vi "raspberry pi red.vi"() -> ()   [LabVIEW 2018]
panel:
  out "Numeric 2":dbl
  out "Waveform Chart 2":dbl(graph)
  out "Humedad":dbl(slide) scale=0.0..100.0
  out "Numeric":dbl
  out "Lectura Raspberry PI":string
  in  "Direcciòn IP":string
  in  "Puerto":i32
  in  "stop":bool
  out "Waveform Chart":dbl(graph)
  out "Temperatura °C":dbl(slide) scale=0.0..100.0
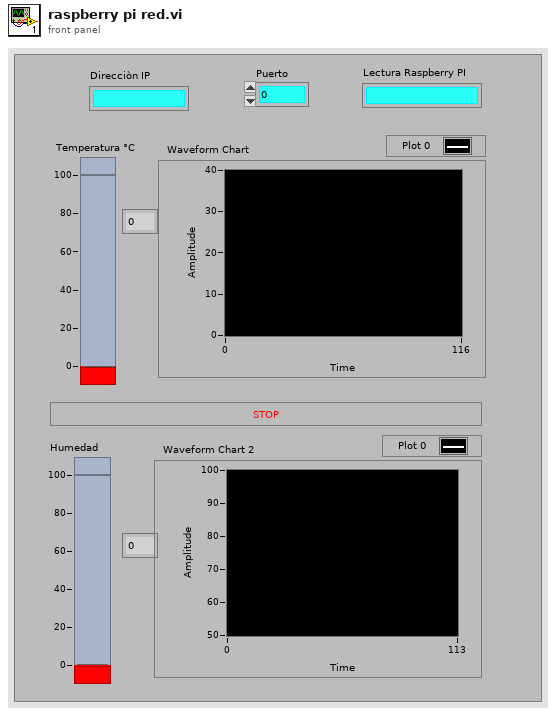
[diagram p1: front panel]
types:
  T1 = enum16{"Standard", "Buffered", "CRLF", "Immediate"}
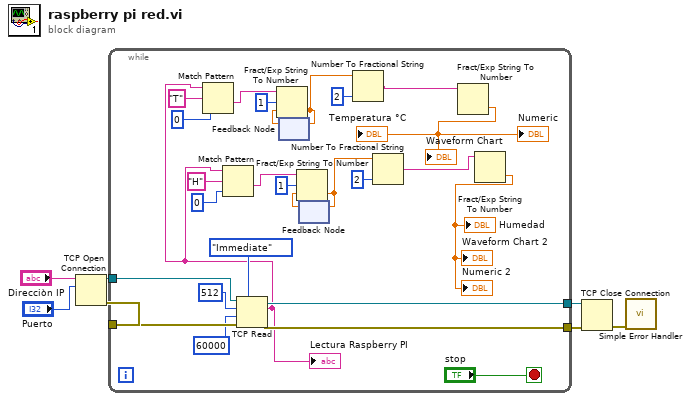
[diagram p0: block diagram]
diagram:
  n1 = TCP Open Connection(address="Direcciòn IP", remote port or service name="Puerto") -> (connection ID=w5:refnum<k5>, error out=w4:errorcluster)  [unwired: 3 in]
  n2 = while {
    tunnel: w5 -> [w33]
    tunnel: w4 -> [w32]
    tunnel: [w31] -> w3
    tunnel: [w30] -> w2
    stop <- "stop" stop-if-true
    n3 = TCP Read(connection ID=w33, bytes to read=512, error in (no error)=w32, 7:T1."Immediate" ("mode (standard)"), 9:60000 ("timeout ms (25000)")) -> (connection ID out=w31:refnum<k5>, data out=w10:string, error out=w30:errorcluster)
    "Lectura Raspberry PI" <- w10
    n4 = Match Pattern(string=w10, regular expression="T", offset (0)=0) -> (after substring=w24:string)  [unwired: 3 out]
    n5 = Match Pattern(string=w10, regular expression="H", offset (0)=0) -> (after substring=w17:string)  [unwired: 3 out]
    n6 = feedback #1() -> (w22:ext)  [unwired: 1 in]
    n7 = Fract/Exp String To Number(string=w24, offset=1, default (0 dbl)=w22) -> (number=w21:ext)  [unwired: 1 in, 1 out]
    n8 = feedback-in #1(w21) -> ()
    n9 = feedback #2() -> (w16:ext)  [unwired: 1 in]
    n10 = Fract/Exp String To Number(string=w17, offset=1, default (0 dbl)=w16) -> (number=w15:ext)  [unwired: 1 in, 1 out]
    n11 = feedback-in #2(w15) -> ()
    n12 = Number To Fractional String(number=w21, precision (6)=i16 2) -> (F-format string=w19:string)  [unwired: 2 in]
    n13 = Number To Fractional String(number=w15, precision (6)=i16 2) -> (F-format string=w8:string)  [unwired: 2 in]
    n14 = Fract/Exp String To Number(string=w19) -> (number=→"Temperatura °C" →"Waveform Chart" →"Numeric":dbl)  [unwired: 3 in, 1 out]
    n15 = Fract/Exp String To Number(string=w8) -> (number=→"Humedad" →"Waveform Chart 2" →"Numeric 2":dbl)  [unwired: 3 in, 1 out]
  }
  n16 = TCP Close Connection(connection ID=w3, error in (no error)=w2) -> (error out=w1:errorcluster)  [unwired: 1 in, 1 out]
  n17 = call <vilib>:"Simple Error Handler.vi"("error in (no error)"=w1) -> ()  [unwired: 4 in, 5 out]
